vi "Database Delete Item.vi"(8 "error in (no error)":errorcluster, 9 "condition":string, 10 "table":string, 11 "object in":refnum<class "Database.lvclass">) -> (0 "error out":errorcluster, 3 "object out":refnum<class "Database.lvclass">)   [LabVIEW 2015, in "Database.lvclass"]
uses:
  Database.lvclass
  Database.lvclass/Database.ctl
  <vilib>/addons/database/Connection.llb/DB Tools Open Connec (String).vi
  <vilib>/addons/database/NI_Database_API.lvlib
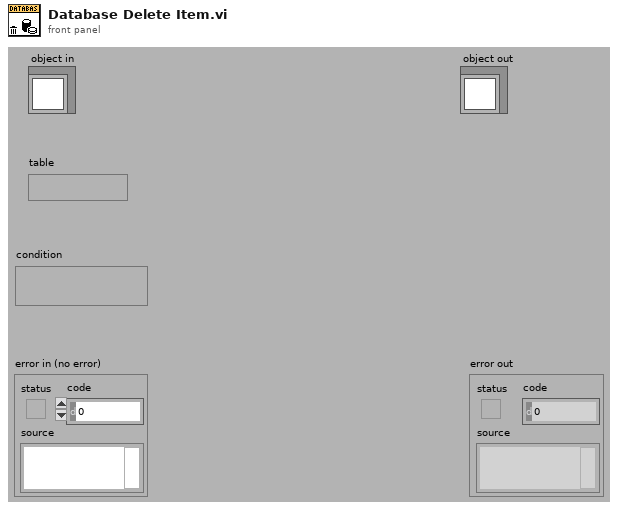
[diagram p1: front panel]
types:
  T1 = typedef "NI_Database_API.lvlib/Conn ObjectReference.ctl" = refnum<k1>
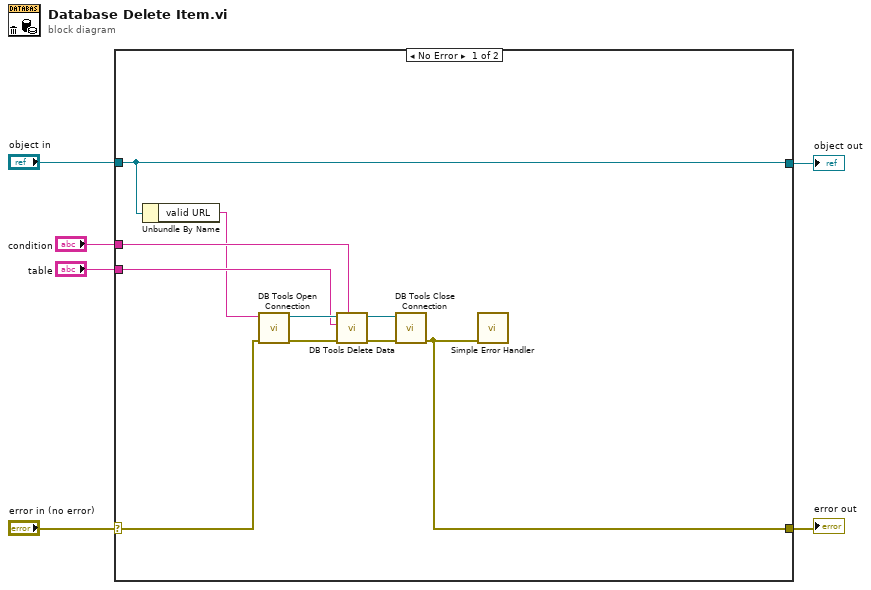
[diagram p0: block diagram]
diagram:
  n1 = case shown="No Error" "error in (no error)" {
    selector: "error in (no error)" -> [w9 w18]
    tunnel: [w12 w18] -> w5
    tunnel: [w8 w17] -> w3
    tunnel: "object in" -> [w8 w17]
    tunnel: "condition" -> [w11 _]
    tunnel: "table" -> [w10 _]
    frame No Error {
      n2 = Unbundle By Name(w8) -> ("valid URL"=w7:string)
      n3 = call-poly <vilib>:"DB Tools Open Connection.vi"("error in (no error)"=w9, "connection information"=w7) -> ("error out"=w15:errorcluster, "connection reference"=w16:T1)  [unwired: 6 in]
      n4 = call <vilib>:"DB Tools Delete Data.vi"("condition"=w11, "error in (no error)"=w15, "table"=w10, "connection reference"=w16) -> ("error out"=w13:errorcluster, "connection reference out"=w14:T1)  [unwired: 6 in]
      n5 = call <vilib>:"DB Tools Close Connection.vi"("error in (no error)"=w13, "connection reference"=w14) -> ("error out"=w12:errorcluster)  [unwired: 5 in]
      n6 = call <vilib>:"Simple Error Handler.vi"("error in (no error)"=w12) -> ()  [unwired: 4 in, 5 out]
    }
    frame Error {
    }
  }
  "error out" <- w5
  "object out" <- w3
